vi "strings to memory.vi"(8 "error in":errorcluster, 11 "1.0.0":T1) -> (0 "error out":errorcluster, 3 "memory hierarchy":T5)   [LabVIEW 2013, in "NISE_CEF_TreeSerializer.lvlib"]
uses:
  NISE_CEF_TreeSerializer.lvlib
  memory hierarchy.ctl
  full hierarchy.ctl
  hierarchy element.ctl
  serializable configuration/NISE_CEF_serializable configuration.lvclass
  flat hierarchy.ctl
  instance data.ctl
  class discovery singleton/class discovery singleton methods.ctl
  class discovery singleton/class discovery singleton.lvlib
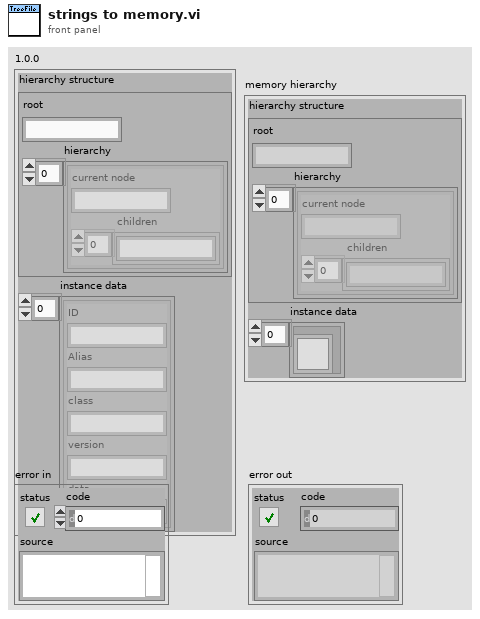
[diagram p1: front panel]
types:
  T1 = typedef "NISE_CEF_TreeSerializer.lvlib/flat hierarchy.ctl" = cluster{"hierarchy structure":T2, "instance data":T4[]}
  T2 = typedef "NISE_CEF_TreeSerializer.lvlib/full hierarchy.ctl" = cluster{"root":string, "hierarchy":T3[]}
  T3 = typedef "NISE_CEF_TreeSerializer.lvlib/hierarchy element.ctl" = cluster{"current node":string, "children":string[]}
  T4 = typedef "NISE_CEF_TreeSerializer.lvlib/instance data.ctl" = cluster{"ID":string, "Alias":string, "class":string, "version":string, "data":string}
  T5 = typedef "NISE_CEF_TreeSerializer.lvlib/memory hierarchy.ctl" = cluster{"hierarchy structure":T2, "instance data":refnum<class "NISE_CEF_serializable configuration.lvclass">[]}
  T6 = typedef "class discovery singleton.lvlib/class discovery singleton methods.ctl" = enum16{"add search paths", "load class by name", "list available classes", "get class path"}
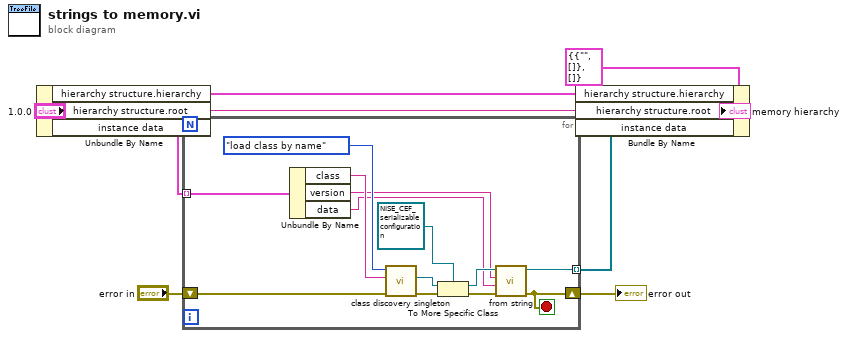
[diagram p0: block diagram]
diagram:
  n1 = Unbundle By Name("1.0.0") -> ("hierarchy structure.hierarchy"=w5:T3[], "hierarchy structure.root"=w6:string, "instance data"=w4:T4[])
  n2 = for {
    tunnel: w4 -> [w22] mode=indexing
    shift-right: [w15] -> w3
    shift-left: "error in" -> [w16]
    tunnel: [w12] -> w1 mode=indexing
    stop <- w15 stop-if-true
    n3 = Unbundle By Name(w22) -> ("class"=w20:string, "version"=w11:string, "data"=w10:string)
    n4 = call "class discovery singleton.vi"("error in"=w16, "Class Name"=w20, "method"=class_discovery_singleton_methods."load class by name") -> ("error out"=w19:errorcluster, "LabVIEW Object"=w18:refnum<class>)  [unwired: 5 in, 2 out]
    n5 = To More Specific Class(target class=refnum<class "NISE_CEF_serializable configuration.lvclass"> refnum ("configuration in"), reference=w18, error in=w19) -> (specific class reference=w13:refnum<class "NISE_CEF_serializable configuration.lvclass">, error out=w14:errorcluster)
    n6 = call-dynamic "from string.vi"("error in"=w14, "data"=w10, "version"=w11, "configuration in"=w13) -> ("error out"=w15:errorcluster, "configuration out"=w12:refnum<class "NISE_CEF_serializable configuration.lvclass">)  [unwired: 6 in]
  }
  "error out" <- w3
  n7 = Bundle By Name(cluster=T5 {"hierarchy structure"={"root"="", "hierarchy"=[]}, "instance data"=[]} ("memory hierarchy"), "hierarchy structure.hierarchy"=w5, "hierarchy structure.root"=w6, "instance data"=w1) -> (→"memory hierarchy":T5)
